vi "Scale Coordinates to Image.vi"(9 "Y":dbl format="%#_13g", 10 "X":dbl format="%#_13g", 11 "Refnum in":T1) -> (3 "Start Point":cluster{"X":i32, "Y":i32})   [LabVIEW 2018]
uses:
  <vilib>/vision/Image Controls.llb/IMAQ Image.ctl
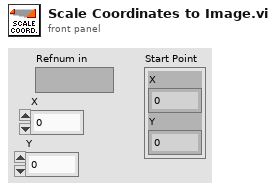
[diagram p1: front panel]
types:
  T1 = typedef "IMAQ Image.ctl" = refnum<image>
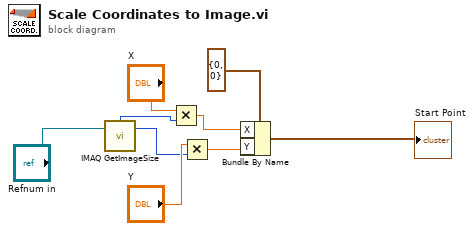
[diagram p0: block diagram]
diagram:
  n1 = call "IMAQ GetImageSize"("Image"="Refnum in") -> ("Y Resolution"=w7:i32, "X Resolution"=w3:i32)  [unwired: 3 in, 1 out]
  n2 = Multiply(x="X", y=w3) -> (x*y=w4:dbl)
  n3 = Multiply(x="Y", y=w7) -> (x*y=w6:dbl)
  n4 = Bundle By Name(cluster=cluster{"X":i32, "Y":i32} {"X"=0, "Y"=0} ("Start Point"), "X"=w4, "Y"=w6) -> (→"Start Point":cluster{"X":i32, "Y":i32})
